vi "Begin.vi"(11 "Image Size":T1=enum."160x120") -> (0 "error out":errorcluster)   [LabVIEW 2012]
doc: "Called before other user functions, this VI is expected to open initial I/O refnums, load in file data, and do all program initialization. Notice that the <B>error out</B> terminal is simply used for data flow. Wiring it to other structures or subVIs ensures that this VI runs first."
uses:
  <vilib>/Rock Robotics/WPI/Camera/WPI_CameraImageSize.ctl
  <vilib>/Rock Robotics/WPI/DriverStation/WPI_DriverStationRobotMode2.ctl
  <vilib>/Rock Robotics/WPI/Joystick/WPI_JoystickDeviceEnum.ctl
  <vilib>/Rock Robotics/SystemInterfaces/DIO/FPGA_DIOPWMChannel.ctl
  <vilib>/Rock Robotics/SystemInterfaces/DIO/FPGA_DIOChannel.ctl
  <vilib>/Rock Robotics/SystemInterfaces/DIO/FPGA_DIORelayChannel.ctl
  <vilib>/Rock Robotics/WPI/Solenoid/WPI_SolenoidChannel.ctl
  Robot Global Data.vi
  <vilib>/Rock Robotics/WPI/MotorControl/WPI_MotorControlOpen Victor.vi
  <vilib>/Rock Robotics/WPI/Solenoid/WPI_SolenoidOpenSingle.vi
  <vilib>/Rock Robotics/WPI/Compressor/WPI_CompressorGetSetRefNum.vi
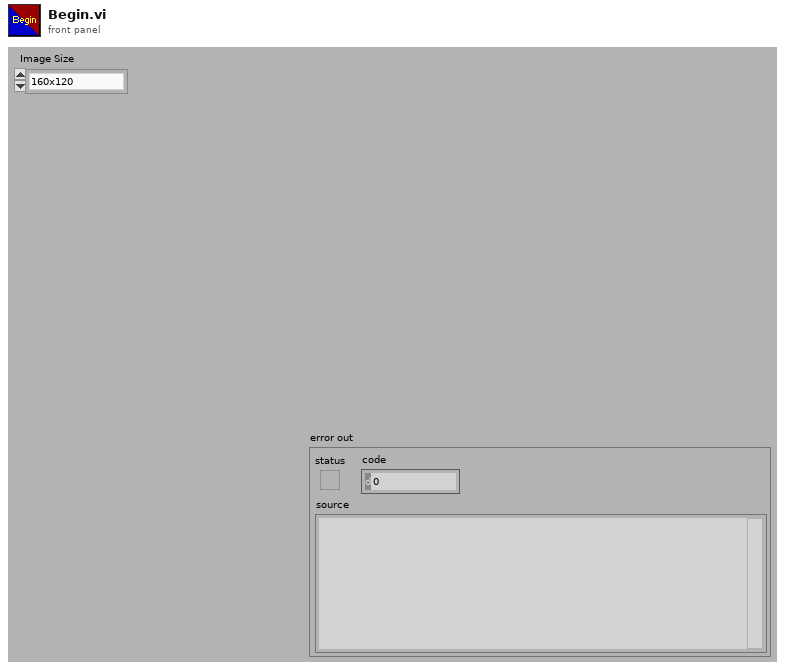
[diagram p1: front panel]
types:
  T1 = typedef "WPI_CameraImageSize.ctl" = enum16{"640x480", "320x240", "160x120"}
  T2 = typedef "WPI_SolenoidChannel.ctl" = enum8{"Solenoid 1", "Solenoid 2", "Solenoid 3", "Solenoid 4", "Solenoid 5", "Solenoid 6", "Solenoid 7", "Solenoid 8", "Invalid"}
  T3 = typedef "FPGA_DIORelayChannel.ctl" = enum8{"Relay 1", "Relay 2", "Relay 3", "Relay 4", "Relay 5", "Relay 6", "Relay 7", "Relay 8", "Invalid"}
  T4 = typedef "FPGA_DIOChannel.ctl" = enum8{"DIO 1", "DIO 2", "DIO 3", "DIO 4", "DIO 5", "DIO 6", "DIO 7", "DIO 8", "DIO 9", "DIO 10", "DIO 11", "DIO 12", "DIO 13", "DIO 14", "Invalid"}
  T5 = typedef "FPGA_DIOPWMChannel.ctl" = enum8{"PWM 1", "PWM 2", "PWM 3", "PWM 4", "PWM 5", "PWM 6", "PWM 7", "PWM 8", "PWM 9", "PWM 10", "Invalid"}
  T6 = typedef "WPI_JoystickDeviceEnum.ctl" = enum16{"USB 1", "USB 2", "USB 3", "USB 4", "Kinect 1", "Kinect 2"}
  T7 = typedef "WPI_DriverStationRobotMode2.ctl" = enum16{"Autonomous Disabled", "Autonomous Enabled", "Teleop Disabled", "Teleop Enabled", "Timeout", "Finish", "Test Disabled", "Test Enabled"}
  T8 = typedef "WPI_CompressorDevRef.ctl" = cluster{"DevStatus":errorcluster, "DigitalInputDevRef":T9, "RelayDevRef":T11}
  T9 = typedef "WPI_DigitalInputDevRef.ctl" = cluster{"DevStatus":errorcluster, "DIO Channel":T4, "Digital Module":T10}
  T10 = typedef "FPGA_TypedefDigitalModule.ctl" = enum16{"Digital Module 1", "Digital Module 2"}
  T11 = typedef "WPI_RelayDevRef.ctl" = cluster{"DevStatus":errorcluster, "Relay Channel":T3, "Digital Module":T10, "Relay Direction":T12}
  T12 = typedef "WPI_RelayDirection.ctl" = enum16{"Both directions", "Forward only", "Reverse only"}
  T13 = typedef "WPI_MotorControlDeviceRef.ctl" = cluster{"DeviceStatus":errorcluster, "Type":enum16{"PWM", "CAN"}, "PWM":cluster{"Digital Module":T10, "PWM Channel":T5, "DeadBand":T14}, "CAN":cluster{"Device Number":u8, "Control Mode":T15, "Semaphore":T16, "Max Vout":dbl}, "Invert":bool, "TransformRef":T17, "InvTransformRef":T17}
  T14 = typedef "WPI_PWMDeadband.ctl" = cluster{"Name":string, "maxPositivePwm":i32, "minPositivePwm":i32, "centerPwm":i32, "maxNegativePwm":i32, "minNegativePwm":i32, "angularRange":u16}
  T15 = typedef "WPI_CANJaguar_ControlMode.ctl" = enum8{"Percent VBus", "Current", "Speed", "Position", "Voltage"}
  T16 = typedef "Semaphore RefNum" = refnum<k1>
  T17 = typedef "WPI_PWMTransform_ConPane.ctl" = refnum<vi>
  T18 = typedef "WPI_SolenoidDevRef.ctl" = cluster{"DevStatus":errorcluster, "Solenoid Module":T19, "Forward Solenoid Channel":T2, "Reverse Solenoid Channel":T2}
  T19 = typedef "FPGA_TypedefSolenoidModule.ctl" = enum16{"Solenoid Module 1", "Solenoid Module 2"}
  T20 = typedef "WPI_JoystickDevRef.ctl" = cluster{"Device":T6}
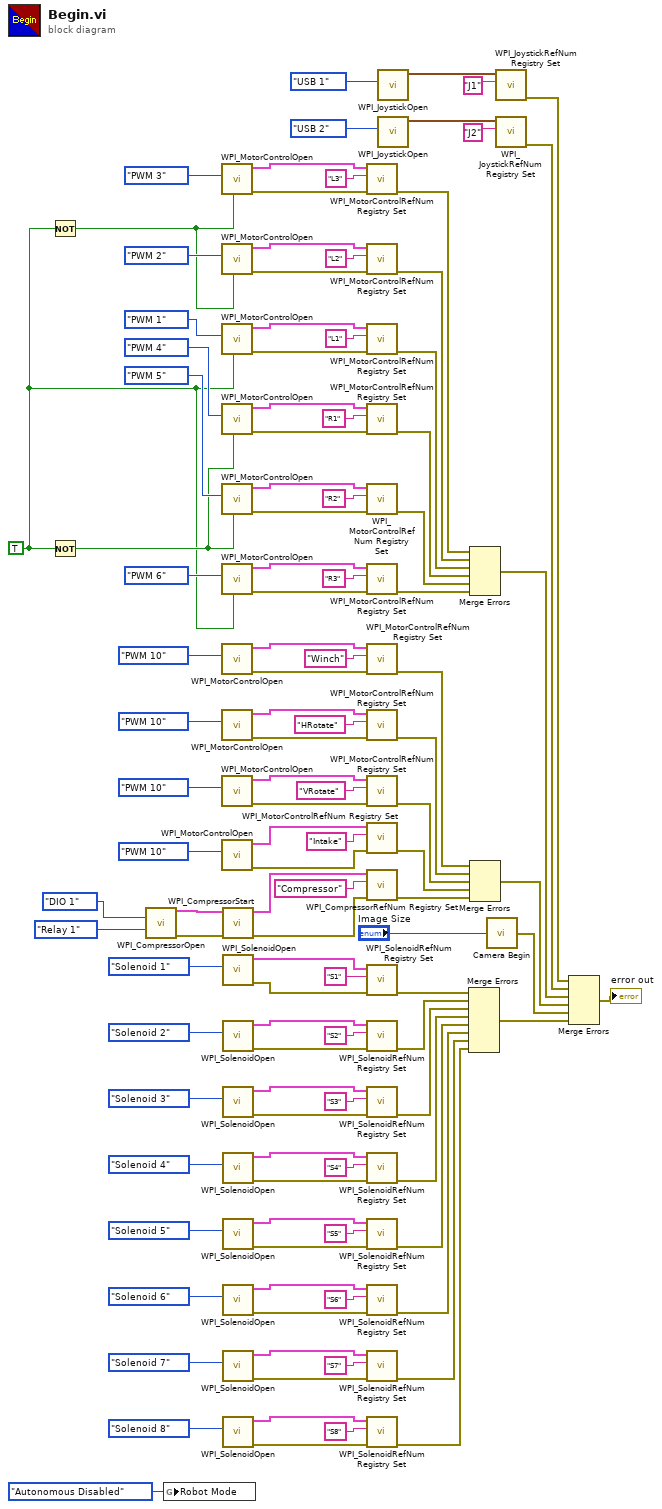
[diagram p0: block diagram]
diagram:
  w42 = TRUE ("Invert")
  n1 = Not(x=w42) -> (.not. x?=w43:bool)
  n2 = Not(x=w42) -> (.not. x?=w44:bool)
  n3 = call <vilib>:"WPI_CompressorOpen.vi"("Pressure Switch DIO Channel"=FPGA_DIOChannel."DIO 1", "Relay Channel"=FPGA_DIORelayChannel."Relay 1") -> ("CompressorDevRef"=w58:T8, "error out"=w59:errorcluster)  [unwired: 12 in]
  n4 = global write "Robot Global Data.vi" "Robot Mode"(WPI_DriverStationRobotMode2."Autonomous Disabled" ("Robot Mode")) -> ()
  n5 = call-poly <vilib>:"WPI_MotorControlOpen.vi"("Invert"=w43, "PWM Channel"=FPGA_DIOPWMChannel."PWM 3") -> ("error out"=w101:errorcluster, "MotorControlDeviceRef"=w100:T13)  [unwired: 8 in]
  n6 = call-poly <vilib>:"WPI_MotorControlOpen.vi"("Invert"=w43, "PWM Channel"=FPGA_DIOPWMChannel."PWM 2") -> ("error out"=w105:errorcluster, "MotorControlDeviceRef"=w104:T13)  [unwired: 8 in]
  n7 = call-poly <vilib>:"WPI_MotorControlOpen.vi"("Invert"=w42, "PWM Channel"=FPGA_DIOPWMChannel."PWM 1") -> ("error out"=w109:errorcluster, "MotorControlDeviceRef"=w108:T13)  [unwired: 8 in]
  n8 = call-poly <vilib>:"WPI_MotorControlOpen.vi"("Invert"=w44, "PWM Channel"=FPGA_DIOPWMChannel."PWM 4") -> ("error out"=w97:errorcluster, "MotorControlDeviceRef"=w96:T13)  [unwired: 8 in]
  n9 = call-poly <vilib>:"WPI_MotorControlOpen.vi"("Invert"=w44, "PWM Channel"=FPGA_DIOPWMChannel."PWM 5") -> ("error out"=w93:errorcluster, "MotorControlDeviceRef"=w92:T13)  [unwired: 8 in]
  n10 = call-poly <vilib>:"WPI_MotorControlOpen.vi"("Invert"=w42, "PWM Channel"=FPGA_DIOPWMChannel."PWM 6") -> ("error out"=w89:errorcluster, "MotorControlDeviceRef"=w88:T13)  [unwired: 8 in]
  n11 = call-poly <vilib>:"WPI_MotorControlOpen.vi"("PWM Channel"=FPGA_DIOPWMChannel."PWM 10") -> ("error out"=w85:errorcluster, "MotorControlDeviceRef"=w84:T13)  [unwired: 9 in]
  n12 = call-poly <vilib>:"WPI_MotorControlOpen.vi"("PWM Channel"=FPGA_DIOPWMChannel."PWM 10") -> ("error out"=w81:errorcluster, "MotorControlDeviceRef"=w80:T13)  [unwired: 9 in]
  n13 = call-poly <vilib>:"WPI_MotorControlOpen.vi"("PWM Channel"=FPGA_DIOPWMChannel."PWM 10") -> ("error out"=w77:errorcluster, "MotorControlDeviceRef"=w76:T13)  [unwired: 9 in]
  n14 = call-poly <vilib>:"WPI_MotorControlOpen.vi"("PWM Channel"=FPGA_DIOPWMChannel."PWM 10") -> ("error out"=w73:errorcluster, "MotorControlDeviceRef"=w72:T13)  [unwired: 9 in]
  n15 = call <vilib>:"WPI_CompressorStart.vi"("error in (no error)"=w59, "CompressorDevRef"=w58) -> ("error out"=w57:errorcluster, "CompressorDevRef"=w56:T8)  [unwired: 8 in]
  n16 = call-poly <vilib>:"WPI_SolenoidOpen.vi"("Solenoid Channel"=WPI_SolenoidChannel."Solenoid 1") -> ("error out"=w41:errorcluster, "SolenoidDevRef"=w40:T18)  [unwired: 9 in]
  n17 = call-poly <vilib>:"WPI_SolenoidOpen.vi"("Solenoid Channel"=WPI_SolenoidChannel."Solenoid 2") -> ("error out"=w37:errorcluster, "SolenoidDevRef"=w36:T18)  [unwired: 9 in]
  n18 = call-poly <vilib>:"WPI_SolenoidOpen.vi"("Solenoid Channel"=WPI_SolenoidChannel."Solenoid 3") -> ("error out"=w33:errorcluster, "SolenoidDevRef"=w32:T18)  [unwired: 9 in]
  n19 = call-poly <vilib>:"WPI_SolenoidOpen.vi"("Solenoid Channel"=WPI_SolenoidChannel."Solenoid 4") -> ("error out"=w29:errorcluster, "SolenoidDevRef"=w28:T18)  [unwired: 9 in]
  n20 = call-poly <vilib>:"WPI_SolenoidOpen.vi"("Solenoid Channel"=WPI_SolenoidChannel."Solenoid 5") -> ("error out"=w25:errorcluster, "SolenoidDevRef"=w24:T18)  [unwired: 9 in]
  n21 = call-poly <vilib>:"WPI_SolenoidOpen.vi"("Solenoid Channel"=WPI_SolenoidChannel."Solenoid 6") -> ("error out"=w21:errorcluster, "SolenoidDevRef"=w20:T18)  [unwired: 9 in]
  n22 = call-poly <vilib>:"WPI_SolenoidOpen.vi"("Solenoid Channel"=WPI_SolenoidChannel."Solenoid 7") -> ("error out"=w17:errorcluster, "SolenoidDevRef"=w16:T18)  [unwired: 9 in]
  n23 = call-poly <vilib>:"WPI_SolenoidOpen.vi"("Solenoid Channel"=WPI_SolenoidChannel."Solenoid 8") -> ("error out"=w13:errorcluster, "SolenoidDevRef"=w12:T18)  [unwired: 9 in]
  n24 = call <vilib>:"WPI_MotorControlRefNum Registry Set.vi"("error in (no error)"=w101, "refnum name"="L3", "MotorControlDevRef"=w100) -> ("error out"=w69:errorcluster)  [unwired: 7 in, 1 out]
  n25 = call <vilib>:"WPI_MotorControlRefNum Registry Set.vi"("error in (no error)"=w105, "refnum name"="L2", "MotorControlDevRef"=w104) -> ("error out"=w68:errorcluster)  [unwired: 7 in, 1 out]
  n26 = call <vilib>:"WPI_MotorControlRefNum Registry Set.vi"("error in (no error)"=w109, "refnum name"="L1", "MotorControlDevRef"=w108) -> ("error out"=w67:errorcluster)  [unwired: 7 in, 1 out]
  n27 = call <vilib>:"WPI_MotorControlRefNum Registry Set.vi"("error in (no error)"=w97, "refnum name"="R1", "MotorControlDevRef"=w96) -> ("error out"=w66:errorcluster)  [unwired: 7 in, 1 out]
  n28 = call <vilib>:"WPI_MotorControlRefNum Registry Set.vi"("error in (no error)"=w93, "refnum name"="R2", "MotorControlDevRef"=w92) -> ("error out"=w65:errorcluster)  [unwired: 7 in, 1 out]
  n29 = call <vilib>:"WPI_MotorControlRefNum Registry Set.vi"("error in (no error)"=w89, "refnum name"="R3", "MotorControlDevRef"=w88) -> ("error out"=w64:errorcluster)  [unwired: 7 in, 1 out]
  n30 = call <vilib>:"WPI_MotorControlRefNum Registry Set.vi"("error in (no error)"=w85, "refnum name"="Winch", "MotorControlDevRef"=w84) -> ("error out"=w63:errorcluster)  [unwired: 7 in, 1 out]
  n31 = call <vilib>:"WPI_MotorControlRefNum Registry Set.vi"("error in (no error)"=w81, "refnum name"="HRotate", "MotorControlDevRef"=w80) -> ("error out"=w62:errorcluster)  [unwired: 7 in, 1 out]
  n32 = call <vilib>:"WPI_MotorControlRefNum Registry Set.vi"("error in (no error)"=w77, "refnum name"="VRotate", "MotorControlDevRef"=w76) -> ("error out"=w61:errorcluster)  [unwired: 7 in, 1 out]
  n33 = call <vilib>:"WPI_MotorControlRefNum Registry Set.vi"("error in (no error)"=w73, "refnum name"="Intake", "MotorControlDevRef"=w72) -> ("error out"=w60:errorcluster)  [unwired: 7 in, 1 out]
  n34 = call <vilib>:"WPI_CompressorRefNum Registry Set.vi"("error in (no error)"=w57, "refnum name"="Compressor", "CompressorDevRef"=w56) -> ("error out"=w52:errorcluster)  [unwired: 7 in, 1 out]
  n35 = call <vilib>:"WPI_SolenoidRefNum Registry Set.vi"("error in (no error)"=w41, "refnum name"="S1", "SolenoidDevRef"=w40) -> ("error out"=w9:errorcluster)  [unwired: 7 in, 1 out]
  n36 = call <vilib>:"WPI_SolenoidRefNum Registry Set.vi"("error in (no error)"=w37, "refnum name"="S2", "SolenoidDevRef"=w36) -> ("error out"=w8:errorcluster)  [unwired: 7 in, 1 out]
  n37 = call <vilib>:"WPI_SolenoidRefNum Registry Set.vi"("error in (no error)"=w33, "refnum name"="S3", "SolenoidDevRef"=w32) -> ("error out"=w7:errorcluster)  [unwired: 7 in, 1 out]
  n38 = call <vilib>:"WPI_SolenoidRefNum Registry Set.vi"("error in (no error)"=w29, "refnum name"="S4", "SolenoidDevRef"=w28) -> ("error out"=w6:errorcluster)  [unwired: 7 in, 1 out]
  n39 = call <vilib>:"WPI_SolenoidRefNum Registry Set.vi"("error in (no error)"=w25, "refnum name"="S5", "SolenoidDevRef"=w24) -> ("error out"=w5:errorcluster)  [unwired: 7 in, 1 out]
  n40 = call <vilib>:"WPI_SolenoidRefNum Registry Set.vi"("error in (no error)"=w21, "refnum name"="S6", "SolenoidDevRef"=w20) -> ("error out"=w4:errorcluster)  [unwired: 7 in, 1 out]
  n41 = call <vilib>:"WPI_SolenoidRefNum Registry Set.vi"("error in (no error)"=w17, "refnum name"="S7", "SolenoidDevRef"=w16) -> ("error out"=w3:errorcluster)  [unwired: 7 in, 1 out]
  n42 = call <vilib>:"WPI_SolenoidRefNum Registry Set.vi"("error in (no error)"=w13, "refnum name"="S8", "SolenoidDevRef"=w12) -> ("error out"=w2:errorcluster)  [unwired: 7 in, 1 out]
  n43 = call <vilib>:"WPI_JoystickOpen.vi"("JoystickDevice"=WPI_JoystickDeviceEnum."USB 1") -> ("JoystickDevRef"=w114:T20)  [unwired: 10 in]
  n44 = call <vilib>:"WPI_JoystickOpen.vi"("JoystickDevice"=WPI_JoystickDeviceEnum."USB 2") -> ("JoystickDevRef"=w111:T20)  [unwired: 10 in]
  n45 = Merge Errors(w9, w8, w7, w6, w5, w4, w3, w2) -> (w1:errorcluster)
  n46 = Merge Errors(w69, w68, w67, w66, w65, w64) -> (w48:errorcluster)
  n47 = Merge Errors(w63, w62, w61, w60, w52) -> (w47:errorcluster)
  n48 = call "Camera Begin.vi"("Image Size"="Image Size") -> ("error out"=w46:errorcluster)
  n49 = call <vilib>:"WPI_JoystickRefNum Registry Set.vi"("refnum name"="J1", "JoystickDevRef"=w114) -> ("error out"=w50:errorcluster)  [unwired: 8 in, 1 out]
  n50 = call <vilib>:"WPI_JoystickRefNum Registry Set.vi"("refnum name"="J2", "JoystickDevRef"=w111) -> ("error out"=w49:errorcluster)  [unwired: 8 in, 1 out]
  n51 = Merge Errors(w50, w49, w48, w47, w46, w1) -> (→"error out":errorcluster)
